vi "sv_Select Harmonics to Visualize.vi"(7 "harmonics to visualize":i32[](array[numeric]), 8 "error in (no error)":errorcluster, 11 "harmonic components":T1(array[cluster]) {"detected amplitude" format="%.2f"; "detected frequency [Hz]" format="%.2f"}) -> (0 "error out":errorcluster, 3 "selected harmonic components":cluster{"frequency [Hz]":dbl, "amplitude":dbl}[](array[cluster]) {"amplitude" format="%.2f"; "frequency [Hz]" format="%.2f"})   [LabVIEW 2017, in "SoundVib_Distortion.lvlib"]
uses:
  <vilib>/addons/Sound and Vibration/svt_Distortion/SoundVib_Distortion.lvlib
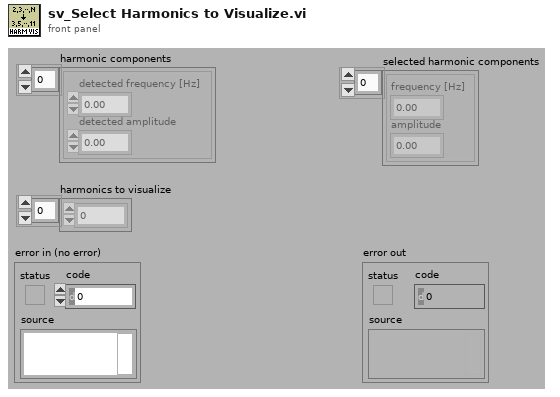
[diagram p1: front panel]
types:
  T1 = cluster{"detected frequency [Hz]":dbl, "detected amplitude":dbl}[]
  T2 = cluster{"detected frequency [Hz]":dbl, "detected amplitude":dbl}
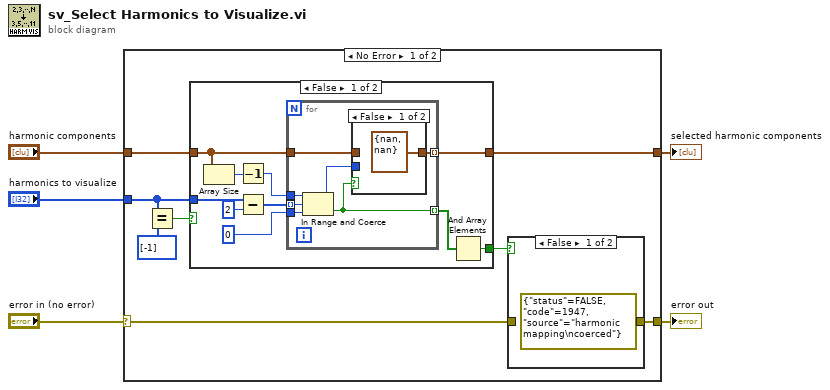
[diagram p0: block diagram]
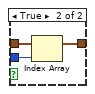
[diagram p3: hidden frame]
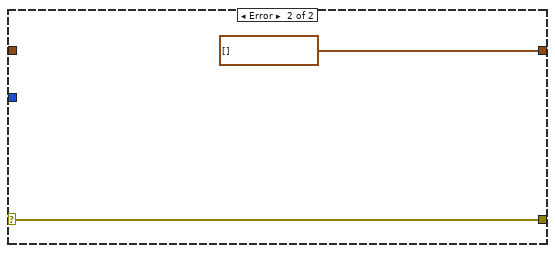
[diagram p5: hidden frame]
diagram:
  n1 = case shown="No Error" "error in (no error)" {
    selector: "error in (no error)" -> [w7 w40]
    tunnel: [w13 T1 []] -> w5
    tunnel: "harmonics to visualize" -> [w11 _]
    tunnel: "harmonic components" -> [w12 _]
    tunnel: [w6 w40] -> w1
    frame No Error {
      n2 = Equal?(x=w11, y=i32[] [-1]) -> (x = y?=w9:bool)
      n3 = case shown="False" w9 {
        selector: w9 -> [_ w37]
        tunnel: [w25 w38] -> w13
        tunnel: w12 -> [w24 w38]
        tunnel: w11 -> [w22 _]
        tunnel: [w20 w37] -> w8
        frame False {
          n4 = Array Size(array=w24) -> (size(s)=w23:i32)
          n5 = Decrement(x=w23) -> (x-1=w18:i32)
          n6 = Subtract(x=w22, y=2) -> (x-y=w19:i32[])
          n7 = for {
            tunnel: [w32] -> w25 mode=indexing
            tunnel: w24 -> [w31]
            tunnel: w19 -> [w28] mode=indexing
            tunnel: w18 -> [w30]
            tunnel: 0 ("lower limit") -> [w29]
            tunnel: [w27] -> w16 mode=indexing
            n8 = In Range and Coerce(upper limit=w30, x=w28, lower limit=w29) -> (coerced(x)=w26:i32, In Range?=w27:bool)
            n9 = case shown="False" w27 {
              tunnel: [T2 {"detected frequency [Hz]"=nan, "detected amplitude"=nan} w36] -> w32
              tunnel: w31 -> [_ w35]
              tunnel: w26 -> [_ w34]
              frame False {
              }
              frame True {
                n10 = Index Array(array=w35, index=w34) -> (element=w36:T2)
              }
            }
          }
          n11 = And Array Elements(Boolean array=w16) -> (logical AND=w20:bool)
        }
        frame True {
        }
      }
      n12 = case shown="False" w8 {
        tunnel: w7 -> [_ w15]
        tunnel: [errorcluster {"status"=FALSE, "code"=1947, "source"="harmonic mapping\ncoerced"} ("error IO") w15] -> w6
        frame False {
        }
        frame True {
        }
      }
    }
    frame Error {
    }
  }
  "selected harmonic components" <- w5
  "error out" <- w1
